vi "SP Read Array.vi"(8 "error in":errorcluster, 11 "Flow Setpoint in":refnum<class "Flow Setpoint.lvclass">) -> (0 "error out":errorcluster, 1 "Changed or First Call?":bool, 2 "Flow SP":dbl[](array[numeric]), 3 "Flow Setpoint out":refnum<class "Flow Setpoint.lvclass">)   [LabVIEW 2023, in "Flow Setpoint.lvclass"]
uses:
  Flow Setpoint.lvclass
  Flow Setpoint.lvclass/Flow Setpoint.ctl
  Parents/Setpoint/Setpoint.lvclass
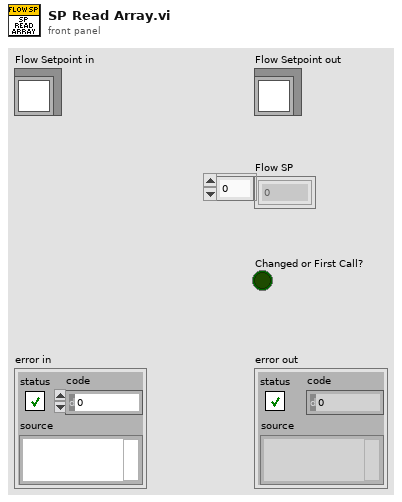
[diagram p1: front panel]
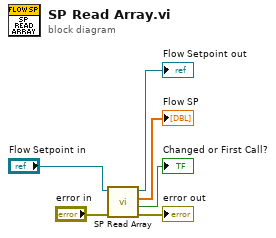
[diagram p0: block diagram]
diagram:
  n1 = call-parent "SP Read Array.vi"("error in"="error in", "Setpoint in"="Flow Setpoint in") -> ("error out"=→"error out":errorcluster, "Changed or First Call?"=→"Changed or First Call?":bool, "Current Setpoint"=→"Flow SP":dbl[], "Setpoint out"=→"Flow Setpoint out":refnum<class "Flow Setpoint.lvclass">)  [unwired: 6 in]
